vi "SendCommandExample.vi"() -> ()   [LabVIEW 2020]
uses:
  <vilib>/httpClient/LabVIEWHTTPClient.lvlib
  <vilib>/wsapi/NI_WebServices.lvlib
panel:
  out "body":string
  out "headers":string
  in  "JSON command":string
  # "(pages 47-50 of user manual)"
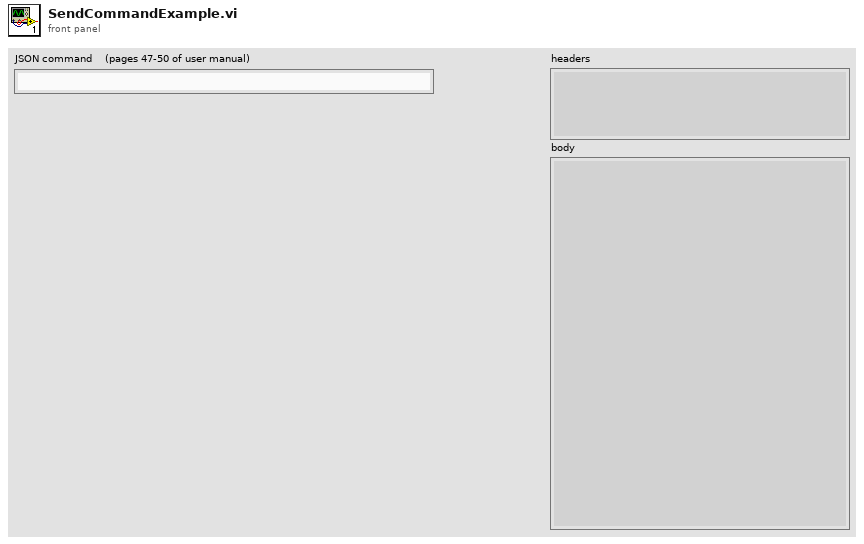
[diagram p1: front panel]
types:
  T1 = typedef "LabVIEWHTTPClient.lvlib/ClientHandle.ctl" = refnum<k1>
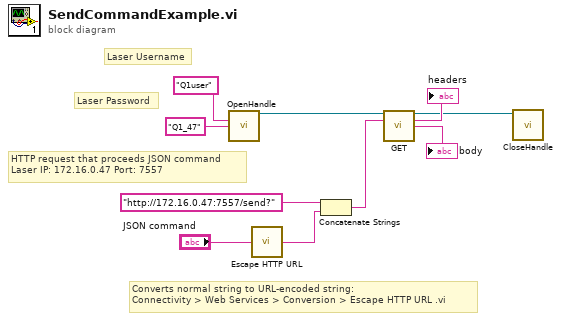
[diagram p0: block diagram]
diagram:
  # "Converts normal string to URL-encoded string:\nConnectivity > Web Services > Conversion > Escape HTTP URL .vi"
  # "HTTP request that proceeds JSON command\nLaser IP: 172.16.0.47 Port: 7557"
  # "Laser Password"
  # "Laser Username"
  n1 = call <vilib>:"OpenHandle.vi"("username"="Q1user", "password"="Q1_47") -> ("client handle out"=w8:T1)  [unwired: 12 in, 1 out]
  n2 = call <vilib>:"Escape HTTP URL.vi"("unescaped string in"="JSON command") -> ("escaped string out"=w2:string)
  n3 = Concatenate Strings("http://172.16.0.47:7557/send?", w2) -> (w4:string)
  n4 = call <vilib>:"GET.vi"("client handle"=w8, "url"=w4) -> ("client handle out"=w1:T1, "headers"=→"headers":string, "body"=→"body":string)  [unwired: 10 in, 1 out]
  n5 = call <vilib>:"CloseHandle.vi"("client handle"=w1) -> ()  [unwired: 14 in, 1 out]
